vi "setWarningAndError.vi"(7 "typeOfWarning":T1, 8 "error in (no error)":errorcluster, 9 "Low":sgl, 10 "High":sgl, 11 "CoolerControler in":refnum<class "CoolerControler.lvclass">) -> (0 "error out":errorcluster, 1 "Low set":sgl, 2 "High set":sgl, 3 "CoolerControler out":refnum<class "CoolerControler.lvclass">)   [LabVIEW 2016, in "CoolerControler.lvclass"]
uses:
  CoolerControler.lvclass
  typedefs/CoolerId.ctl
  typeOfWarning.ctl
  SerialCommand/CoolerSerialCommand.lvclass
  typedefs/dataUnit.ctl
  typedefs/CoolerCommands.ctl
panel:
  in  "id":T2=1
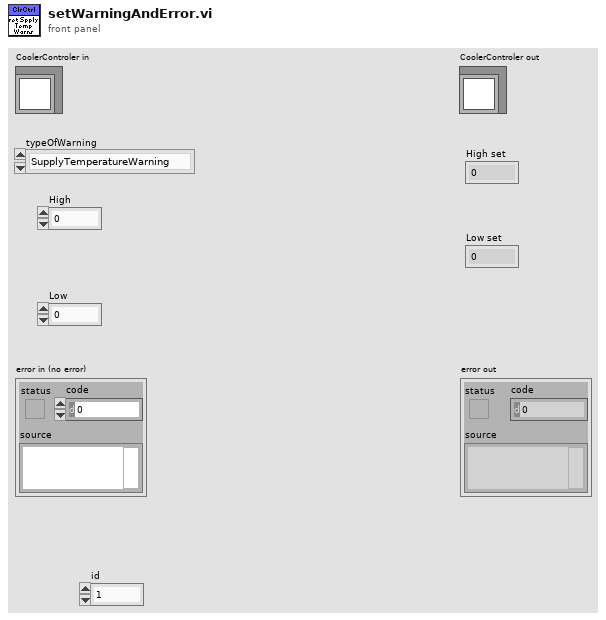
[diagram p1: front panel]
types:
  T1 = typedef "typeOfWarning.ctl" = enum16{"SupplyTemperatureWarning", "AmbientTemperatureWarning", "lowFlowWarning", "SupplyTemperatureAlarm", "AmbientTemperatureAlarm", "lowFlowAlarm"}
  T2 = typedef "CoolerId.ctl" = u16
  T3 = typedef "dataUnit.ctl" = enum16{"temperature", "flow", "current", "PID", "fanSpeed", "time", "PWM", "TEDriveLevel", "Number"}
  T4 = typedef "CoolerCommands.ctl" = enum16{"None", "SetExternSensorStatus", "SetChillerStatus", "SetControlSensor", "SetControlTemperature", "SetHighSupplyTempWarning", "SetLowSupplyTemperatureWarning", "SetHighAmbientTemperatureWarning", "SetLowAmbienTemperatureWarning", "SetLowProcessFlowWarning", "SetHighSupplyTemperatureAlarm", "SetLowSupplyTemperatureAlarm", "SetHighAmbientTemperatureAlarm", "SetLowAmbientTemperatureAlarm", "SetLowProcessFlowAlarm"}
  T5 = typedef "response.ctl" = cluster{"deviceId":string, "commandNumber":string, "errorActive":bool, "commandName":string, "responseData":string, "checkSum":string}
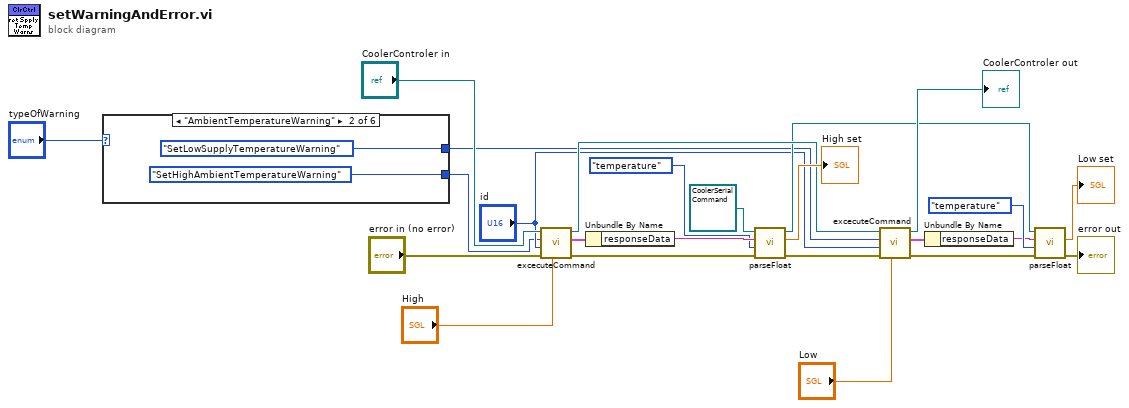
[diagram p0: block diagram]
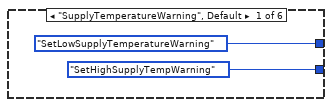
[diagram p2: hidden frame]
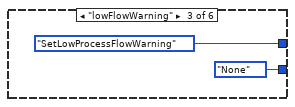
[diagram p3: hidden frame]
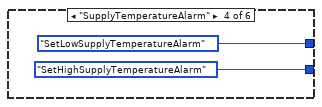
[diagram p4: hidden frame]
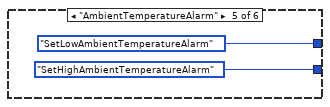
[diagram p5: hidden frame]
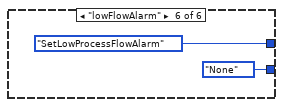
[diagram p6: hidden frame]
diagram:
  n1 = case shown="\"AmbientTemperatureWarning\"" "typeOfWarning" {
    tunnel: [CoolerCommands."SetHighSupplyTempWarning" ("CoolerCommand") CoolerCommands."SetHighAmbientTemperatureWarning" ("CoolerCommand") CoolerCommands."None" ("CoolerCommand") CoolerCommands."SetHighSupplyTemperatureAlarm" ("CoolerCommand") CoolerCommands."SetHighAmbientTemperatureAlarm" ("CoolerCommand") CoolerCommands."None" ("CoolerCommand")] -> w4
    tunnel: [CoolerCommands."SetLowSupplyTemperatureWarning" ("CoolerCommand") CoolerCommands."SetLowSupplyTemperatureWarning" ("CoolerCommand") CoolerCommands."SetLowProcessFlowWarning" ("CoolerCommand") CoolerCommands."SetLowSupplyTemperatureAlarm" ("CoolerCommand") CoolerCommands."SetLowAmbientTemperatureAlarm" ("CoolerCommand") CoolerCommands."SetLowProcessFlowAlarm" ("CoolerCommand")] -> w3
    frame "SupplyTemperatureWarning", Default {
    }
    frame "AmbientTemperatureWarning" {
    }
    frame "lowFlowWarning" {
    }
    frame "SupplyTemperatureAlarm" {
    }
    frame "AmbientTemperatureAlarm" {
    }
    frame "lowFlowAlarm" {
    }
  }
  n2 = call "excecuteCommand.vi"("inputValue"="High", "error in (no error)"="error in (no error)", "id"="id", "CoolerCommand"=w4, "CoolerControler in"="CoolerControler in") -> ("error out"=w19:errorcluster, "response out"=w20:T5, "CoolerControler out"=w12:refnum<class "CoolerControler.lvclass">)  [unwired: 4 in]
  n3 = Unbundle By Name(w20) -> ("responseData"=w24:string)
  n4 = call "parseFloat.vi"("error in (no error)"=w19, "unit"=dataUnit."temperature", "commandData"=w24, "CoolerSerialCommand in"=refnum<class "CoolerSerialCommand.lvclass"> refnum) -> ("error out"=w9:errorcluster, "value"=→"High set":sgl, "CoolerSerialCommand out"=w10:refnum<class "CoolerSerialCommand.lvclass">)  [unwired: 4 in, 1 out]
  n5 = call "excecuteCommand.vi"("inputValue"="Low", "error in (no error)"=w9, "id"="id", "CoolerCommand"=w3, "CoolerControler in"=w12) -> ("error out"=w16:errorcluster, "response out"=w15:T5, "CoolerControler out"=→"CoolerControler out":refnum<class "CoolerControler.lvclass">)  [unwired: 4 in]
  n6 = Unbundle By Name(w15) -> ("responseData"=w13:string)
  n7 = call "parseFloat.vi"("error in (no error)"=w16, "unit"=dataUnit."temperature", "commandData"=w13, "CoolerSerialCommand in"=w10) -> ("error out"=→"error out":errorcluster, "value"=→"Low set":sgl)  [unwired: 4 in, 2 out]
